vi "Write Single Register.vi"(8 "error in (no error)":errorcluster, 9 "register value":u16, 10 "address":u16, 11 "device data model in":refnum<class "ICPCON ET Data Model.lvclass">) -> (0 "error out":errorcluster, 3 "device data model out":refnum<class "ICPCON ET Data Model.lvclass">)   [LabVIEW 2021, in "ICPCON ET Data Model.lvclass"]
doc: "Writes the value of a single holding register."
uses:
  ICPCON ET Data Model.lvclass
  ICPCON ET Data Model.lvclass/ICPCON ET Data Model.ctl
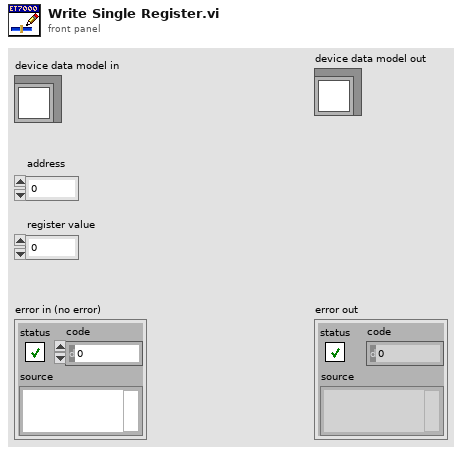
[diagram p1: front panel]
types:
  T1 = typedef "ICPCON ET Data Model.lvclass/Data Model.ctl" = cluster{"UTC":u64, "DI":bool[], "DO":bool[], "IR":u16[], "HR":u16[], "ES":u8}
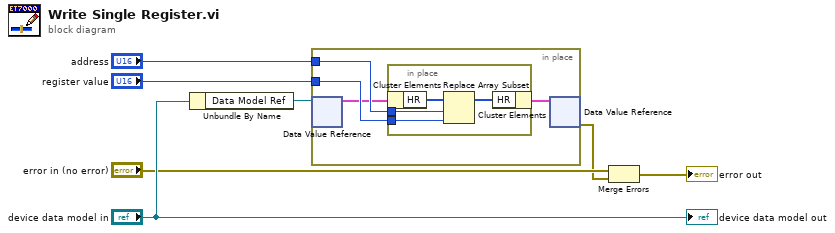
[diagram p0: block diagram]
diagram:
  n1 = Unbundle By Name("device data model in") -> ("Data Model Ref"=w2:refnum<data-value>)
  n2 = in-place {
    in-place-border: "address" -> [w11]
    in-place-border: "register value" -> [w10]
    n3 = in-place-dvr #1(w2) -> (w9:T1)  [unwired: 1 out]
    n4 = in-place {
      in-place-border: w11 -> [w15]
      in-place-border: w10 -> [w14]
      n5 = in-place-cluster #2(w9) -> ("HR"=w13:u16[])
      n6 = Replace Array Subset(array=w13, new element=w14, index=w15) -> (w12:u16[])
      n7 = in-place-cluster #2("HR"=w12) -> (w8:T1)
    }
    n8 = in-place-dvr #1(w8) -> (w1:errorcluster)  [unwired: 1 out]
  }
  n9 = Merge Errors("error in (no error)", w1) -> (→"error out":errorcluster)
  "device data model out" <- "device data model in"
